vi "AutoDistance.vi"(5 "Auto":bool, 7 "Mode":T1, 8 "Slowdown":dbl format="%#_13g", 9 "Brake":dbl format="%#_13g", 10 "DesiredDistance":dbl format="%#_13g", 11 "CurrentDistance":dbl format="%#_13g") -> (1 "TankDriveRight":dbl, 2 "TankDriveLeft":dbl, 3 "Finished":bool=TRUE)   [LabVIEW 2013]
doc: "Determines the motor inputs needed for the left and right sides of tank drive to reach the distance setpoint.\n-Mode: fullspeed (i.e. floor it until the robot gets there) or linear (linear relation between distance to go and motor input).\n-DesiredDistance: the setpoint distance\n-CurrentDistance: the current distance to the target\n-Brake: the minimum distance from the setpoint the robot needs to be in order to brake\n-Slowdown: the maximum distance from the setpoint at which the robot can go full speed\n-Auto, true if auto is active, false if teleop is active."
uses:
  AutoAlignMode.ctl
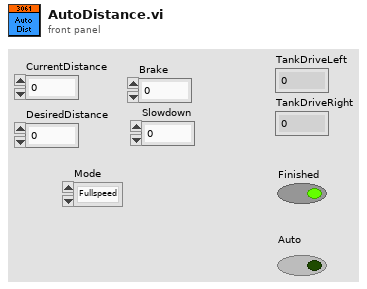
[diagram p1: front panel]
types:
  T1 = typedef "AutoAlignMode.ctl" = enum16{"Fullspeed", "Linear"}
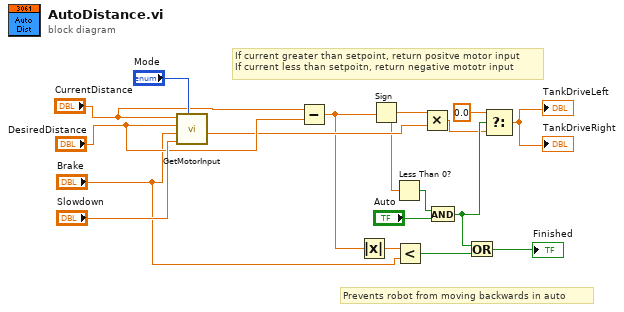
[diagram p0: block diagram]
diagram:
  # "Prevents robot from moving backwards in auto"
  # "If current greater than setpoint, return positve motor input\nIf current less than setpoitn, return negative mototr input"
  n1 = call "GetMotorInput.vi"("Mode"="Mode", "Slowdown"="Slowdown", "Brake"="Brake", "Setpoint"="DesiredDistance", "Current"="CurrentDistance") -> ("MotorInput"=w13:dbl)  [unwired: 6 in]
  n2 = Subtract(x="CurrentDistance", y="DesiredDistance") -> (x-y=w12:dbl)
  n3 = Absolute Value(x=w12) -> (abs(x)=w11:dbl)
  n4 = Sign(1:w12) -> (0:w5:dbl)
  n5 = Less Than 0?(x=w5) -> (x < 0?=w6:bool)
  n6 = Less?(x=w11, y="Brake") -> (x < y?=w8:bool)
  n7 = Multiply(x=w5, y=w13) -> (x*y=w1:dbl)
  n8 = And(x=w6, y="Auto") -> (x .and. y?=w3:bool)
  n9 = Or(x=w3, y=w8) -> (x .or. y?=→"Finished":bool)
  n10 = Select(t=0.0 ("f"), s=w3, f=w1) -> (s? t:f=→"TankDriveLeft" →"TankDriveRight":dbl)
